vi "Visit.vi"(8 "error in (no error)":errorcluster, 10 "Equipment":refnum<class "Equipment.lvclass">, 11 "reference in":refnum<class "EquipmentVisitor.lvclass">) -> (0 "error out":errorcluster, 3 "reference out":refnum<class "EquipmentVisitor.lvclass">)   [LabVIEW 2020, in "EquipmentVisitor.lvclass"]
uses:
  EquipmentVisitor.lvclass
  Equipment_class/Equipment.lvclass
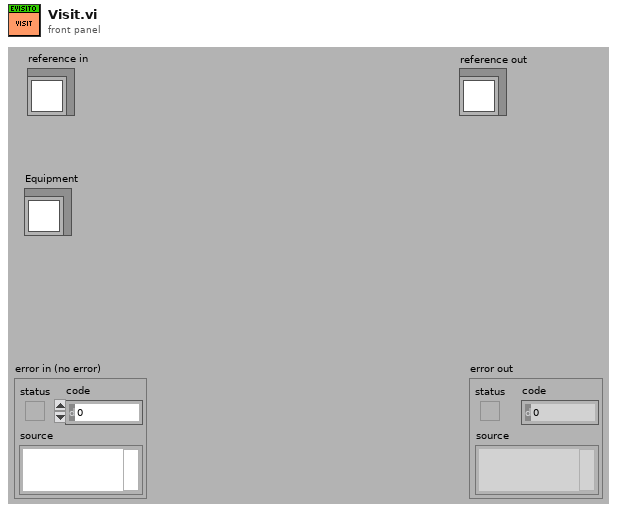
[diagram p1: front panel]
types:
  T1 = typedef "EquipmentVisitor.lvclass/ObjectAttributes.ctl" = cluster{"Equipment":refnum<class "Equipment.lvclass">}
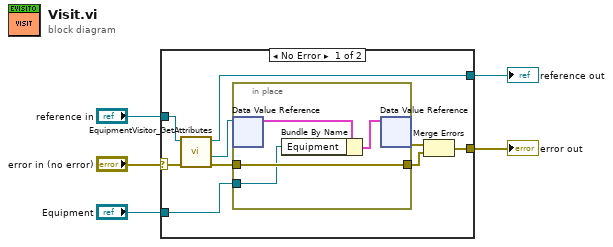
[diagram p0: block diagram]
diagram:
  n1 = case shown="No Error" "error in (no error)" {
    selector: "error in (no error)" -> [w13 w20]
    tunnel: [w10 w20] -> w4
    tunnel: [w11 w19] -> w2
    tunnel: "reference in" -> [w14 w19]
    tunnel: "Equipment" -> [w6 _]
    frame No Error {
      n2 = call "EquipmentVisitor_GetAttributes.vi"("error in (no error)"=w13, "reference in"=w14) -> ("error out"=w8:errorcluster, "DataRef"=w9:refnum<data-value>, "reference out"=w11:refnum<class "EquipmentVisitor.lvclass">)  [unwired: 6 in, 1 out]
      n3 = in-place {
        in-place-border: w8 -> [w17]
        in-place-border: [w17] -> w7
        in-place-border: w6 -> [w15]
        n4 = in-place-dvr #1(w9) -> (w16:T1)  [unwired: 1 out]
        n5 = Bundle By Name(cluster=w16, "Equipment"=w15) -> (w18:T1)
        n6 = in-place-dvr #1(w18) -> (w12:errorcluster)  [unwired: 1 out]
      }
      n7 = Merge Errors(w12, w7) -> (w10:errorcluster)
    }
    frame Error {
    }
  }
  "error out" <- w4
  "reference out" <- w2
